vi "Do Request.vi"(7 "Processing In":refnum<class "Processing.lvclass">, 11 "InfoController in":refnum<class "InfoController.lvclass">) -> (0 "error out":errorcluster, 5 "Processing":refnum<class "Processing.lvclass">)   [LabVIEW 2020, in "Vecto.lvlib" / "InfoController.lvclass"]
uses:
  InfoController.lvclass
  lv-http-server/HTTP Server/Processing/Processing.lvclass
  Info Segment.ctl
  lv-http-server/HTTP Server/Processing/Processing.lvclass/Processing.ctl
  InfoService/NodeStatus.lvclass
  C:/dev/lv20CE/relink/lv-http-server/HTTP Server/Service/Service.lvclass
  VectoService/VectoInfo.lvclass
  lv-http-util/HTTP Utils/Response/Response.lvclass
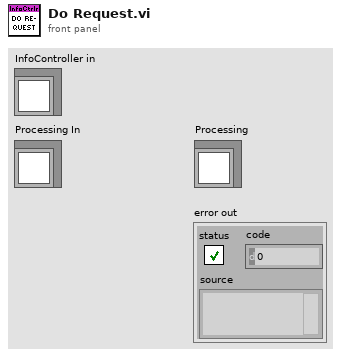
[diagram p1: front panel]
types:
  T1 = typedef "Vecto.lvlib/InfoController.lvclass/Info Segment.ctl" = enum16{"UNKNOWN", "node", "status", "health"}
  T2 = typedef "Vecto.lvlib/Node Info.ctl" = cluster{"Name":string, "ID":u32, "Status":string, "SWVersion":string, "ConfigVersion":string, "Tasks":T3[]}
  T3 = typedef "VectoConfig.lvlib/Task Info.ctl" = cluster{"Name":string, "Status":string}
  T4 = typedef "Vecto.lvlib/Vecto Info.ctl" = cluster{"NodeID":i32, "IP":u32, "Connections":T5[]}
  T5 = typedef "Vecto.lvlib/Connection Info.ctl" = cluster{"Name":string, "Type":T6, "RXCount":i32, "TXCount":i32, "Connected":bool, "RemoteIP":u32, "RemotePort":u16, "LocalPort":u16, "Node ID":u32}
  T6 = typedef "Vecto.lvlib/Connection Type.ctl" = enum16{"TCP", "Telemetry", "Discovery", "HTTP"}
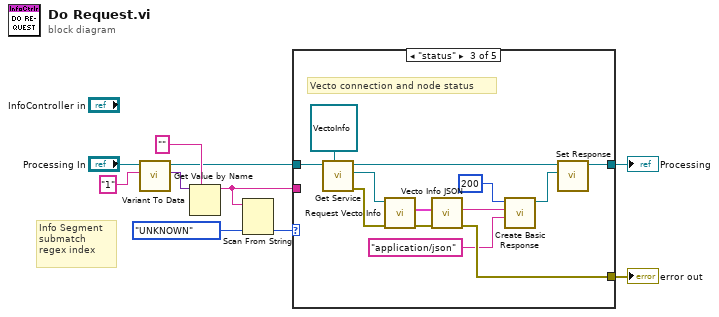
[diagram p0: block diagram]
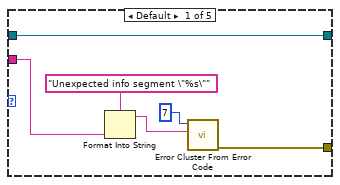
[diagram p2: hidden frame]
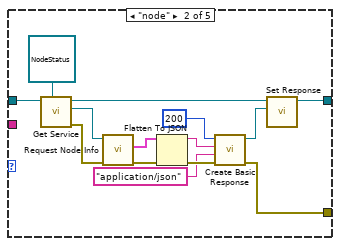
[diagram p3: hidden frame]
diagram:
  # "Info Segment submatch regex index"
  n1 = call "Get Value by Name.vi"("Name"="1", "Processing in"="Processing In") -> ("Value"=w8:variant, "Processing out"=w6:refnum<class "Processing.lvclass">)  [unwired: 7 in, 1 out]
  n2 = Variant To Data(type="", Variant=w8) -> (data=w3:string)  [unwired: 1 in, 1 out]
  n3 = Scan From String(input string=w3, default 1=Info_Segment."UNKNOWN" ("Info Segment")) -> (output 1=w4:T1)  [unwired: 3 in, 3 out]
  n4 = case shown="\"status\"" w4 {
    tunnel: w6 -> [w11 w30 w35 w44 w45]
    tunnel: w3 -> [w14 _ _ _ _]
    tunnel: [w12 w17 w43 _ _] -> w2
    tunnel: [w11 w18 w31 w44 w45] -> w1
    frame Default {
      n5 = Format Into String(format string="Unexpected info segment \"%s\"", w14) -> (resulting string=w13:string)  [unwired: 2 in, 1 out]
      n6 = call <vilib>:"Error Cluster From Error Code.vi"("error message (\"\")"=w13, "error code (0)"=7) -> ("error out"=w12:errorcluster)  [unwired: 7 in]
    }
    frame "node" {
      n7 = call "Get Service.vi"("Service Type"=refnum<class "NodeStatus.lvclass"> refnum ("Vecto.lvlib:InfoService.lvclass"), "Processing in"=w30) -> ("error out"=w28:errorcluster, "Service"=w27:refnum<class "NodeStatus.lvclass">, "Processing out"=w20:refnum<class "Processing.lvclass">)  [unwired: 7 in]
      n8 = call "Request Node Info.vi"("error in (no error)"=w28, "InfoService in"=w27) -> ("error out"=w25:errorcluster, "Node Info"=w26:T2)  [unwired: 7 in, 1 out]
      n9 = Flatten To JSON(anything=w26, error in (no error)=w25) -> (JSON string=w23:string, 11:w24:errorcluster)  [unwired: 1 in]
      n10 = call "Create Basic Response.vi"("error in (no error)"=w24, "Content-Type (text/plain)"="application/json", "Payload"=w23, "Status Code"=u16 200) -> ("error out"=w17:errorcluster, "Response out"=w19:refnum<class "Response.lvclass">)  [unwired: 6 in]
      n11 = call "Set Response.vi"("Response"=w19, "Processing in"=w20) -> ("Processing out"=w18:refnum<class "Processing.lvclass">)  [unwired: 9 in]
    }
    frame "status" {
      # "Vecto connection and node status"
      n12 = call "Get Service.vi"("Service Type"=refnum<class "VectoInfo.lvclass"> refnum ("Vecto.lvlib:VectoService.lvclass"), "Processing in"=w35) -> ("error out"=w41:errorcluster, "Service"=w40:refnum<class "VectoInfo.lvclass">, "Processing out"=w37:refnum<class "Processing.lvclass">)  [unwired: 7 in]
      n13 = call "Request Vecto Info.vi"("error in (no error)"=w41, "VectoService in"=w40) -> ("error out"=w33:errorcluster, "Vecto Info"=w34:T4)  [unwired: 7 in, 1 out]
      n14 = call "Vecto Info JSON.vi"("error in (no error)"=w33, "Vecto Info"=w34) -> ("error out"=w43:errorcluster, "JSON string"=w32:string)  [unwired: 8 in]
      n15 = call "Create Basic Response.vi"("Content-Type (text/plain)"="application/json", "Payload"=w32, "Status Code"=u16 200) -> ("Response out"=w36:refnum<class "Response.lvclass">)  [unwired: 7 in, 1 out]
      n16 = call "Set Response.vi"("Response"=w36, "Processing in"=w37) -> ("Processing out"=w31:refnum<class "Processing.lvclass">)  [unwired: 9 in]
    }
    frame "health" {
      # "Reports as much health information as is available, task rates, data rates, disk usage, cpu usage, etc"
    }
    frame "UNKNOWN" {
    }
  }
  "error out" <- w2
  "Processing" <- w1
